vi "Create.vi"(8 "error in (no error)":errorcluster) -> (0 "error out":errorcluster, 3 "CodeCoverage out":refnum<class "Code Coverage.lvclass">)   [LabVIEW 2017, in "Code Coverage.lvclass"]
doc: "Creates a new application instance for code coverage analysis."
uses:
  Code Coverage.lvclass
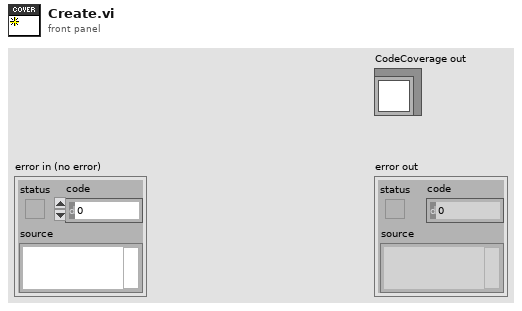
[diagram p1: front panel]
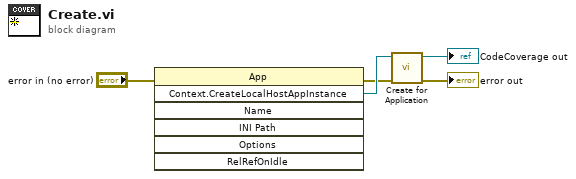
[diagram p0: block diagram]
diagram:
  n1 = invoke class="App" method="Context.CreateLocalHostAppInstance"(error in="error in (no error)") -> (error out=w3:errorcluster, "Create Context"=w4:refnum<vi>)  [unwired: 6 in, 5 out]
  n2 = call "Create for Application.vi"("error in (no error)"=w3, "Application"=w4) -> ("error out"=→"error out":errorcluster, "CodeCoverage out"=→"CodeCoverage out":refnum<class "Code Coverage.lvclass">)  [unwired: 8 in]
